vi "Frecuencia.vi"(8 "error in (no error)":errorcluster, 10 "Frecuencia":dbl, 11 "Measurement gg in":refnum<class "Measurement gg.lvclass">) -> (0 "error out":errorcluster, 3 "Measurement gg out":refnum<class "Measurement gg.lvclass">)   [LabVIEW 2020, in "Measurement gg.lvlib" / "Measurement gg.lvclass"]
uses:
  Measurement gg.lvclass
  Measurement gg.lvclass/Measurement gg.ctl
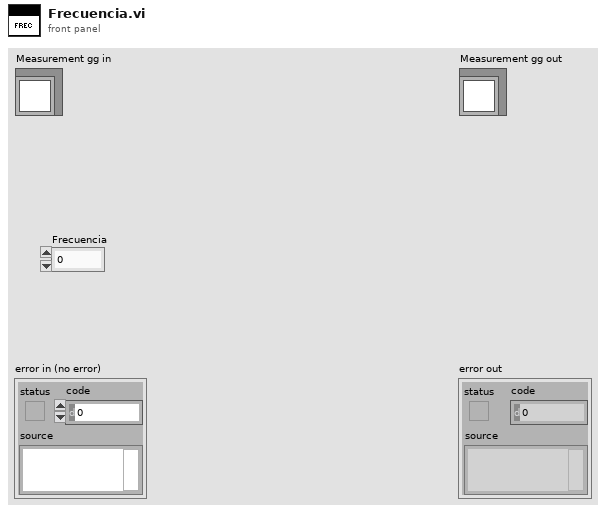
[diagram p1: front panel]
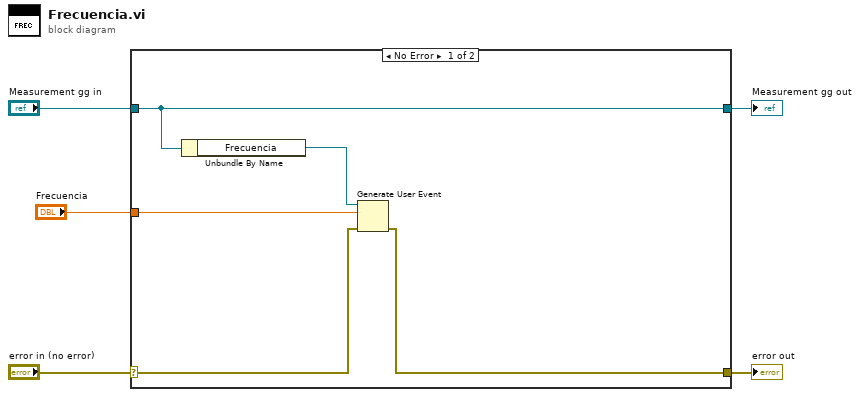
[diagram p0: block diagram]
diagram:
  n1 = case shown="No Error" "error in (no error)" {
    selector: "error in (no error)" -> [w8 w12]
    tunnel: [w7 w12] -> w4
    tunnel: [w10 w11] -> w2
    tunnel: "Measurement gg in" -> [w10 w11]
    tunnel: "Frecuencia" -> [w6 _]
    frame No Error {
      n2 = Unbundle By Name(w10) -> ("Frecuencia"=w9:refnum<user-event>)
      n3 = Generate User Event(user event=w9, event data cluster=w6, error in=w8) -> (error out=w7:errorcluster)  [unwired: 1 in, 1 out]
    }
    frame Error {
    }
  }
  "error out" <- w4
  "Measurement gg out" <- w2
